vi "PH_Beckhoff_Application.declare analog MA01 InputTags.vi"() -> (0 "Analog Inputs":T3, 1 "Description":string)   [LabVIEW 2014, in "PH_Beckhoff_Application.lvlib"]
uses:
  PH_Beckhoff_Application.lvlib
  PH_Beckhoff/PH_Beckhoff.Analog Inputs.ctl
  PH_Beckhoff/PH_Beckhoff.Scaling Type.ctl
  PH_Beckhoff/PH_Beckhoff.lvlib
panel:
  in  "Analog Input Value":T2
  out "Right Size?":bool
  # "Let this VI run to check the size!"
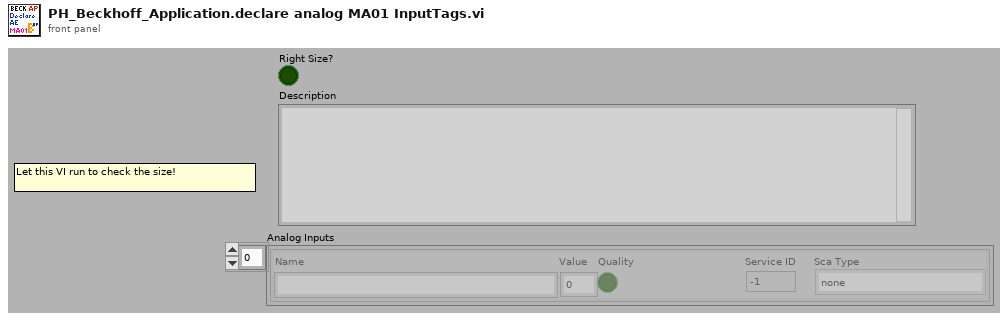
[diagram p1: front panel]
types:
  T1 = typedef "PH_Beckhoff.lvlib/PH_Beckhoff.Scaling Type.ctl" = enum16{"none", "0 ... 15 Bit -> 0 ... 5", "0 ... 15 Bit -> 0 ... 10", "0 ... 15 Bit -> 0 ... 25", "0 ... 15 Bit -> 4 ... 20", "0 ... 15 Bit -> 0 ... 1", "0 ... 15 Bit -> 0 ... 20000", "0 ... 15 Bit -> 0 ... 24000"}
  T2 = cluster{"Name":string, "Value":u32, "Quality":bool, "Service ID":i32, "Sca Type":T1}
  T3 = typedef "PH_Beckhoff.lvlib/PH_Beckhoff.Analog Inputs.ctl" = cluster{"Name":string, "Value":u32, "Quality":bool, "Service ID":i32, "Sca Type":T1}[]
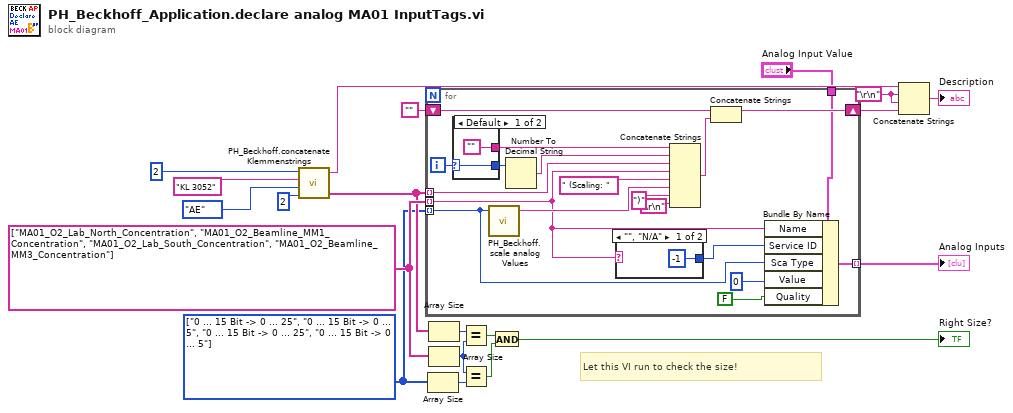
[diagram p0: block diagram]
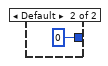
[diagram p2: hidden frame]
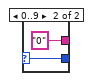
[diagram p3: hidden frame]
diagram:
  w2 = T1[] [enum."0 ... 15 Bit -> 0 ... 25", enum."0 ... 15 Bit -> 0 ... 5", enum."0 ... 15 Bit -> 0 ... 25", enum."0 ... 15 Bit -> 0 ... 5"] items=["none", "0 ... 15 Bit -> 0 ... 5", "0 ... 15 Bit -> 0 ... 10", "0 ... 15 Bit -> 0 ... 25", "0 ... 15 Bit -> 4 ... 20", "0 ... 15 Bit -> 0 ... 1", "0 ... 15 Bit -> 0 ... 20000", "0 ... 15 Bit -> 0 ... 24000"]
  w10 = string[] ["MA01_O2_Lab_North_Concentration", "MA01_O2_Beamline_MM1_Concentration", "MA01_O2_Lab_South_Concentration", "MA01_O2_Beamline_MM3_Concentration"]
  w18 = "\r\n"
  # "Let this VI run to check the size!"
  n1 = call "PH_Beckhoff.concatenate Klemmenstrings.vi"("# of In- or Outputs"=2, "Type"=enum16{"AE", "AA", "DE", "DA"}."AE", "Klemmenname"="KL 3052", "Quantity"=2) -> ("concatenated string array"=w9:string[], "\"<Type>: <Quantity> x <Klemmenname>\""=w8:string)  [unwired: 1 out]
  n2 = for {
    tunnel: w10 -> [w27] mode=indexing
    tunnel: w9 -> [w35] mode=indexing
    shift-right: [w32] -> w19
    shift-left: "" -> [w31]
    tunnel: w2 -> [w22] mode=indexing
    tunnel: [w23] -> w3 mode=indexing
    tunnel: "Analog Input Value" -> [w21]
    i -> [w39]
    n3 = case shown="Default" w39 {
      selector: w39 -> [w42 w45]
      tunnel: [w42 w45] -> w38
      tunnel: ["" "0"] -> w37
      frame Default {
      }
      frame 0..9 {
      }
    }
    n4 = call "PH_Beckhoff.scale analog Values.vi"("Sca Type"=w22) -> ("Scaling"=w30:string)  [unwired: 2 in, 2 out]
    n5 = Number To Decimal String(number=w38) -> (decimal integer string=w36:string)  [unwired: 1 in]
    n6 = case shown="\"\", \"N/A\"" w27 {
      tunnel: [-1 0] -> w26
      frame "", "N/A" {
      }
      frame Default {
      }
    }
    n7 = Concatenate Strings(w37, w36, w35, w27, " (Scaling: " ("string"), w30, ")" ("string"), "\r\n") -> (w33:string)
    n8 = Concatenate Strings(w31, w33) -> (w32:string)
    n9 = Bundle By Name(cluster=w21, "Name"=w27, "Service ID"=w26, "Sca Type"=w22, "Value"=u32 0, "Quality"=FALSE) -> (w23:T2)
  }
  "Analog Inputs" <- w3
  n10 = Array Size(array=w2) -> (size(s)=w6:i32)
  n11 = Array Size(array=w9) -> (size(s)=w16:i32)
  n12 = Array Size(array=w10) -> (size(s)=w7:i32)
  n13 = Equal?(x=w16, y=w7) -> (x = y?=w15:bool)
  n14 = Equal?(x=w7, y=w6) -> (x = y?=w4:bool)
  n15 = And(x=w15, y=w4) -> (x .and. y?=→"Right Size?":bool)
  n16 = Concatenate Strings(w8, w18, w18, w19) -> (→"Description":string)
